vi "BarcodeSN.vi"(8 "error in (no error)":errorcluster, 11 "VISA resource name":refnum<visa-resource-name>) -> (0 "error out":errorcluster, 3 "Barcode":string)   [LabVIEW 2019]
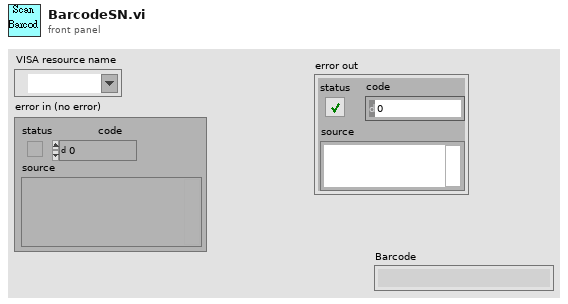
[diagram p1: front panel]
types:
  T1 = enum16{"Open", "Send", "Recieve", "Recieve cmd", "Close"}
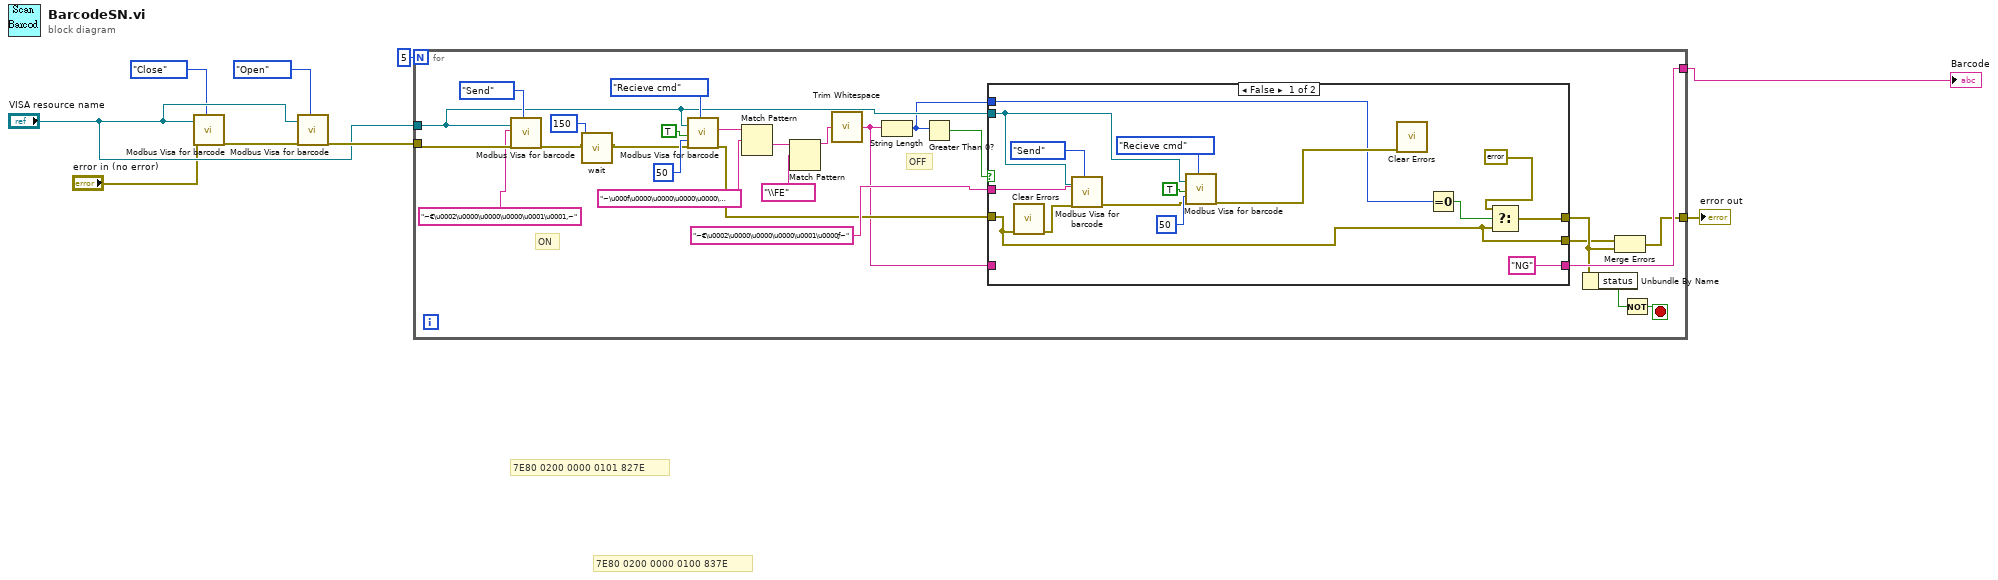
[diagram p0: block diagram]
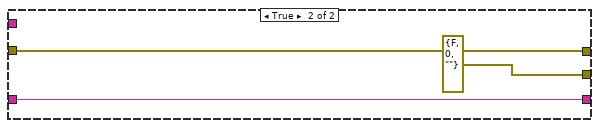
[diagram p2: hidden frame]
diagram:
  # "7E80 0200 0000 0100 837E"
  # "7E80 0200 0000 0101 827E"
  n1 = call "Modbus Visa for barcode .vi"("VISA resource name"="VISA resource name", "error in (no error)"="error in (no error)", "VisaAction"=T1."Close") -> ("error out"=w4:errorcluster)  [unwired: 15 in, 1 out]
  n2 = call "Modbus Visa for barcode .vi"("VISA resource name"="VISA resource name", "error in (no error)"=w4, "VisaAction"=T1."Open") -> ("error out"=w8:errorcluster)  [unwired: 15 in, 1 out]
  n3 = for {
    N: 5 -> [_]
    tunnel: w8 -> [w35]
    tunnel: "VISA resource name" -> [w27]
    tunnel: [w10] -> w6
    tunnel: [w16] -> w1
    stop <- w32 stop-if-true
    # "OFF"
    # "ON"
    n4 = call "Modbus Visa for barcode .vi"("VISA resource name"=w27, "Cmd"="~€\u0002\u0000\u0000\u0000\u0001\u0001‚~", "error in (no error)"=w35, "VisaAction"=T1."Send") -> ("error out"=w14:errorcluster)  [unwired: 14 in, 1 out]
    n5 = call "wait.vi"("error in"=w14, "wait(ms)"=u32 150) -> ("error out"=w13:errorcluster)  [unwired: 9 in]
    n6 = call "Modbus Visa for barcode .vi"("VISA resource name"=w27, "TimeOut"=TRUE, "Time(0.1)"=u32 50, "error in (no error)"=w13, "VisaAction"=T1."Recieve cmd") -> ("read string"=w22:string, "error out"=w24:errorcluster)  [unwired: 13 in]
    n7 = Match Pattern(string=w22, regular expression="~\u000f\u0000\u0000\u0000\u0000\u0000\u000f~" ("trimmed string")) -> (after substring=w21:string)  [unwired: 1 in, 3 out]
    n8 = Match Pattern(string=w21, regular expression="\\FE") -> (before substring=w20:string)  [unwired: 1 in, 3 out]
    n9 = call <vilib>:"Trim Whitespace.vi"("string"=w20) -> ("trimmed string"=w17:string)  [unwired: 1 in]
    n10 = String Length(string=w17) -> (length=w18:i32)
    n11 = Greater Than 0?(x=w18) -> (x > 0?=w34:bool)
    n12 = case shown="False" w34 {
      tunnel: w24 -> [w36 w52]
      tunnel: [w47 w52] -> w12
      tunnel: w27 -> [w41 _]
      tunnel: "~€\u0002\u0000\u0000\u0000\u0001\u0000ƒ~" ("Cmd") -> [w40 _]
      tunnel: w18 -> [w38 _]
      tunnel: w17 -> [_ w53]
      tunnel: ["NG" ("trimmed string") w53] -> w16
      tunnel: [w36 errorcluster {"status"=FALSE, "code"=0, "source"=""} ("error out")] -> w11
      frame False {
        n13 = call <vilib>:"Clear Errors.vi"("error in (no error)"=w36) -> ("error out"=w50:errorcluster)  [unwired: 5 in, 1 out]
        n14 = call "Modbus Visa for barcode .vi"("VISA resource name"=w41, "Cmd"=w40, "error in (no error)"=w50, "VisaAction"=T1."Send") -> ("error out"=w42:errorcluster)  [unwired: 14 in, 1 out]
        n15 = call "Modbus Visa for barcode .vi"("VISA resource name"=w41, "TimeOut"=TRUE, "Time(0.1)"=u32 50, "error in (no error)"=w42, "VisaAction"=T1."Recieve cmd") -> ("error out"=w39:errorcluster)  [unwired: 13 in, 1 out]
        n16 = call <vilib>:"Clear Errors.vi"("error in (no error)"=w39) -> ()  [unwired: 5 in, 2 out]
        n17 = Equal To 0?(x=w38) -> (x = 0?=w48:bool)
        n18 = Select(t=errorcluster {"status"=TRUE, "code"=13602, "source"="讀取條碼異常"} ("error constant"), s=w48, f=w36) -> (s? t:f=w47:errorcluster)
      }
      frame True {
      }
    }
    n19 = Unbundle By Name(w12) -> ("status"=w33:bool)
    n20 = Merge Errors(w11, w12) -> (w10:errorcluster)
    n21 = Not(x=w33) -> (.not. x?=w32:bool)
  }
  "error out" <- w6
  "Barcode" <- w1
